vi "Read Slot Settings.vi"(8 "error in (no error)":errorcluster, 11 "RSI Module in":refnum<class "RSI Module.lvclass">) -> (0 "error out":errorcluster, 2 "Slot Settings":T1, 3 "RSI Module out":refnum<class "RSI Module.lvclass">)   [LabVIEW 2020, in "Modules.lvlib" / "RSI Module.lvclass"]
uses:
  RSI Module.lvclass
  Slot Settings.ctl
  RSI Module.lvclass/RSI Module.ctl
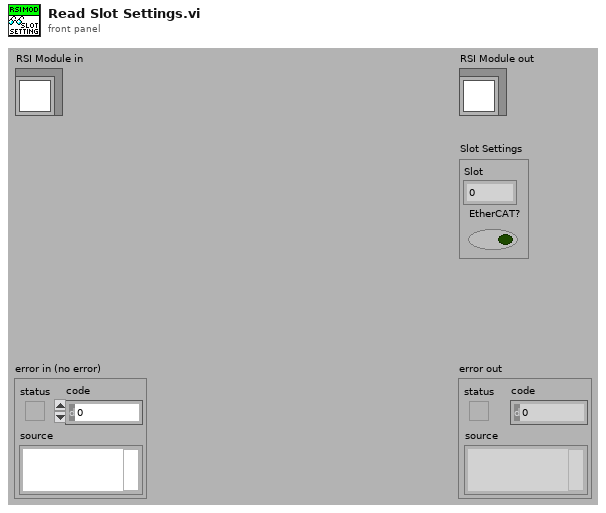
[diagram p1: front panel]
types:
  T1 = typedef "Modules.lvlib/RSI Module.lvclass/Slot Settings.ctl" = cluster{"Slot":u32, "EtherCAT?":bool}
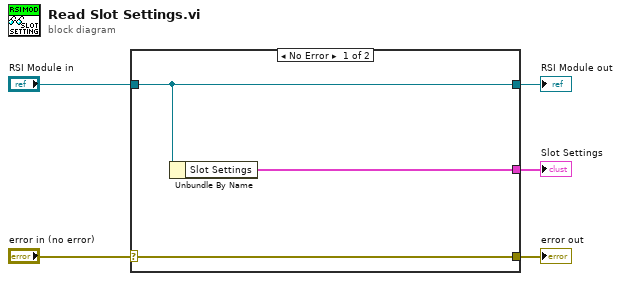
[diagram p0: block diagram]
diagram:
  n1 = case shown="No Error" "error in (no error)" {
    selector: "error in (no error)" -> [w8 w9]
    tunnel: [w8 w9] -> w4
    tunnel: [w7 w10] -> w2
    tunnel: "RSI Module in" -> [w7 w10]
    tunnel: [w6 _] -> w1
    frame No Error {
      n2 = Unbundle By Name(w7) -> ("Slot Settings"=w6:T1)
    }
    frame Error {
    }
  }
  "error out" <- w4
  "RSI Module out" <- w2
  "Slot Settings" <- w1
